vi "Calc Measruement Details.vi"(11 "Measurement properties":T1={"Measurement ID"=enum."1 signal, 1 ADC, 1 PJVS", "Description"="3 phase, 3 ADC, 1 PJVS", "Switching matrix M"=[], "Signal frequency  (Hz)"=50.0, "Maximal signal amplitude (V)"=0.0, "PRs (s)"=1.0, "PRe (s)"=50.0, "MRs (s)"=0.0, "MRe (s)"=0.0, "Set PJVS frequency (Hz)"=50.0, "PJVS reference voltages (1 period, V)"=[], "Requiested PJVS steps"=10, "Sampling f (Hz)"=0.0, "Trigger mode"=enum."Trigger every MX switch", "Timing matrix (periods)"=[], "Record length (multiples of M)"=1, "Calculated"={"Triggers to next path (line of sequence)"=[], "Record samples"=0, "Sample indexes of switches"=[], "PRs (samples)"=0, "PRe (samples)"=0, "MRs (samples)"=0, "MRe (samples)"=0, "Trigger frequency  (Hz)"=50.0, "Measurement druation (s)"=0.0, "Samples per step"=0.0, "QPMX Sequence"=[]}, "No of digitizers"=0, "No of transducers"=0, "Transducer corrections"=[]} {"Calculated"."Trigger frequency  (Hz)" format="%#_6p"; "Record length (multiples of M)" min=1 step=1; "PJVS reference voltages (1 period, V)" format="%.9g"; "MRe (s)" format="%#_4p"; "MRs (s)" format="%#_4p"; "PRe (s)" format="%#.4p"; "PRs (s)" format="%#_4p"}) -> (3 "Measurement properties out":T1={"Measurement ID"=enum."1 signal, 1 ADC, 1 PJVS", "Description"="3 phase, 3 ADC, 1 PJVS", "Switching matrix M"=[], "Signal frequency  (Hz)"=50.0, "Maximal signal amplitude (V)"=0.0, "PRs (s)"=1.0, "PRe (s)"=50.0, "MRs (s)"=0.0, "MRe (s)"=0.0, "Set PJVS frequency (Hz)"=50.0, "PJVS reference voltages (1 period, V)"=[], "Requiested PJVS steps"=10, "Sampling f (Hz)"=0.0, "Trigger mode"=enum."Trigger every MX switch", "Timing matrix (periods)"=[], "Record length (multiples of M)"=1, "Calculated"={"Triggers to next path (line of sequence)"=[], "Record samples"=0, "Sample indexes of switches"=[], "PRs (samples)"=0, "PRe (samples)"=0, "MRs (samples)"=0, "MRe (samples)"=0, "Trigger frequency  (Hz)"=50.0, "Measurement druation (s)"=0.0, "Samples per step"=0.0, "QPMX Sequence"=[]}, "No of digitizers"=0, "No of transducers"=0, "Transducer corrections"=[]} {"Calculated"."Trigger frequency  (Hz)" format="%#_6p"; "Record length (multiples of M)" min=1 step=1; "PJVS reference voltages (1 period, V)" format="%.9g"; "MRe (s)" format="%#_4p"; "MRs (s)" format="%#_4p"; "PRe (s)" format="%#.4p"; "PRs (s)" format="%#_4p"})   [LabVIEW 2020]
uses:
  Type definitions/Measuement properties.ctl
  Type definitions/Measurement ID.ctl
  Type definitions/Trigger mode.ctl
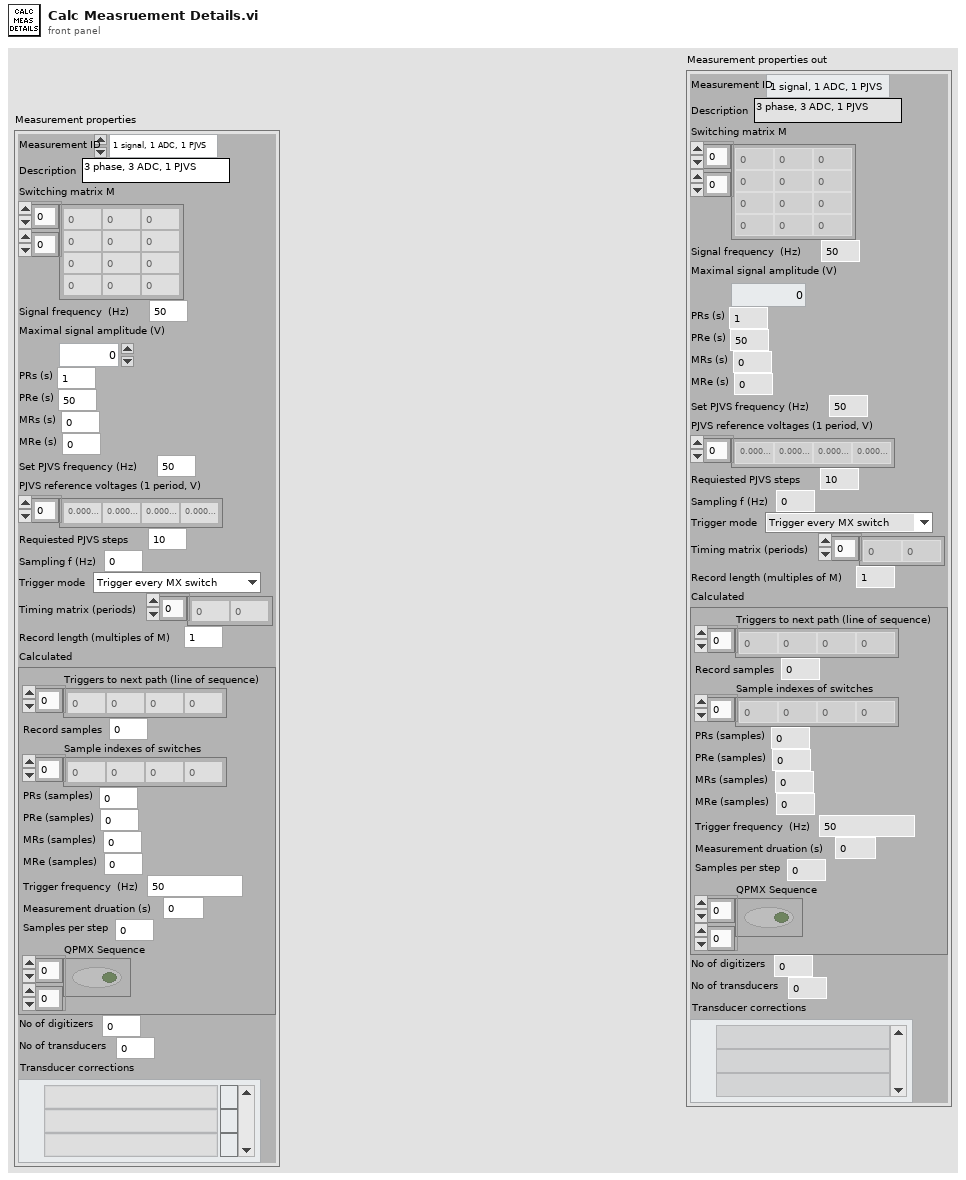
[diagram p1: front panel]
types:
  T1 = typedef "Measuement properties.ctl" = cluster{"Measurement ID":T2, "Description":string, "Switching matrix M":i32[][], "Signal frequency  (Hz)":dbl, "Maximal signal amplitude (V)":dbl, "PRs (s)":dbl, "PRe (s)":dbl, "MRs (s)":dbl, "MRe (s)":dbl, "Set PJVS frequency (Hz)":dbl, "PJVS reference voltages (1 period, V)":dbl[], "Requiested PJVS steps":u32, "Sampling f (Hz)":dbl, "Trigger mode":T3, "Timing matrix (periods)":i32[], "Record length (multiples of M)":u32, "Calculated":cluster{"Triggers to next path (line of sequence)":u32[], "Record samples":u32, "Sample indexes of switches":u32[], "PRs (samples)":i32, "PRe (samples)":i32, "MRs (samples)":i32, "MRe (samples)":i32, "Trigger frequency  (Hz)":dbl, "Measurement druation (s)":dbl, "Samples per step":dbl, "QPMX Sequence":bool[][]}, "No of digitizers":u32, "No of transducers":u32, "Transducer corrections":path[]}
  T2 = typedef "Measurement ID.ctl" = enum16{"Manual setup", "1 signal, 1 ADC, 1 PJVS", "1 phase (U, I), 1 ADC, 1 PJVS", "1 phase (U, I), 2 ADC, 1 PJVS", "1 phase (U, I), 3 ADC, 1 PJVS", "3 phases (U1..3, I1..3), 3 ADC, 1 PJVS"}
  T3 = typedef "Trigger mode.ctl" = enum16{"Trigger every MX switch", "Trigger every sample"}
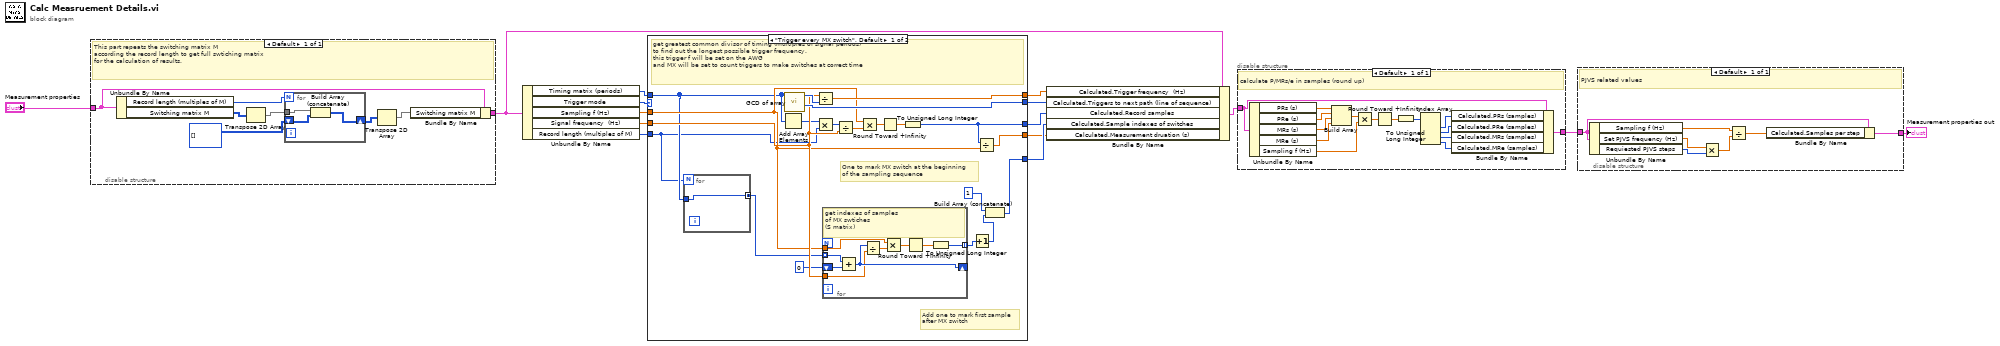
[diagram p0: block diagram]
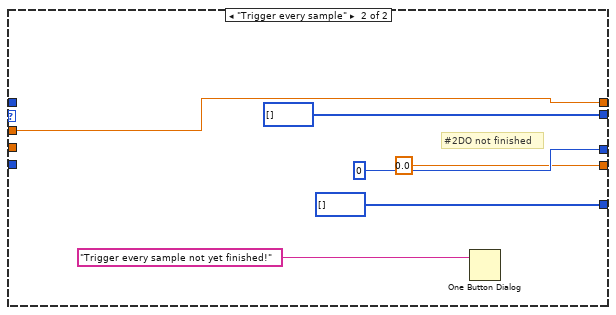
[diagram p2: hidden frame]
diagram:
  n1 = disable-structure shown="Default" {
    disable-tunnel: "Measurement properties" -> [w22]
    disable-tunnel: [w21] -> w1
    frame Enabled {
      # "This part repeats the switching matrix M\naccording the record length to get full swtiching matrix\nfor the calculation of results."
      n2 = Unbundle By Name(w22) -> ("Record length (multiples of M)"=w23:u32, "Switching matrix M"=w19:i32[][])
      n3 = Transpose 2D Array(2D array=w19) -> (transposed array=w18:i32[][])
      n4 = for {
        N: w23 -> [_]
        tunnel: w18 -> [w26]
        shift-right: [w24] -> w17
        shift-left: i32[][] [] ("Switching matrix M") -> [w25]
        n5 = Build Array (concatenate)(w26, w25) -> (w24:i32[][])
      }
      n6 = Transpose 2D Array(2D array=w17) -> (transposed array=w16:i32[][])
      n7 = Bundle By Name(cluster=w22, "Switching matrix M"=w16) -> (w21:T1)
    }
  }
  n8 = Unbundle By Name(w1) -> ("Timing matrix (periods)"=w7:i32[], "Trigger mode"=w15:T3, "Sampling f (Hz)"=w13:dbl, "Signal frequency  (Hz)"=w12:dbl, "Record length (multiples of M)"=w6:u32)
  n9 = case shown="\"Trigger every MX switch\", Default" w15 {
    tunnel: [w46 w62] -> w14
    tunnel: w13 -> [w36 w62]
    tunnel: w12 -> [w40 _]
    tunnel: w7 -> [w29 _]
    tunnel: [w44 u32[] [] ("Divisors")] -> w11
    tunnel: [w37 u32 0] -> w10
    tunnel: [w33 u32[] []] -> w9
    tunnel: w6 -> [w28 _]
    tunnel: [w35 0.0] -> w5
    frame "Trigger every MX switch", Default {
      # "Add one to mark first sample\nafter MX switch"
      # "One to mark MX switch at the beginning\nof the sampling sequence"
      # "get greatest common divisor of timing (multiples of signal periods)\nto find out the longest possible trigger frequency. \nthis trigger f will be set on the AWG\nand MX will be set to count triggers to make switches at correct time"
      n10 = for {
        N: w28 -> [_]
        tunnel: w29 -> [w47]
        tunnel: [w47] -> w27 mode=concatenating
      }
      n11 = Add Array Elements(numeric array=w29) -> (sum=w39:i32)
      n12 = call "GCD of array.vi"("Array"=w29) -> ("Divisors"=w44:u32[], "GCD"=w45:u32)  [unwired: 9 in]
      n13 = Divide(x=w40, y=w45) -> (x/y=w46:dbl)
      n14 = Multiply(x=w39, y=w28) -> (x*y=w38:u32)
      n15 = for {
        tunnel: w27 -> [w56] mode=indexing
        shift-right: [w51] -> _
        shift-left: u32 0 ("y") -> [w55]
        tunnel: w40 -> [w50]
        tunnel: [w49] -> w32 mode=indexing
        tunnel: w36 -> [w48]
        # "get indexes of samples\nof MX swtiches\n(S matrix)"
        n16 = Add(x=w56, y=w55) -> (x+y=w51:u32)
        n17 = Divide(x=w51, y=w50) -> (x/y=w52:dbl)
        n18 = Multiply(x=w48, y=w52) -> (x*y=w53:dbl)
        n19 = Round Toward +Infinity(x=w53) -> (ceil(x): smallest int >= x=w54:dbl)
        n20 = To Unsigned Long Integer(number=w54) -> (unsigned 32bit integer=w49:u32)
      }
      n21 = Divide(x=w38, y=w40) -> (x/y=w43:dbl)
      n22 = Multiply(x=w36, y=w43) -> (x*y=w42:dbl)
      n23 = Round Toward +Infinity(x=w42) -> (ceil(x): smallest int >= x=w41:dbl)
      n24 = To Unsigned Long Integer(number=w41) -> (unsigned 32bit integer=w37:u32)
      n25 = Increment(x=w32) -> (x+1=w31:u32[])
      n26 = Divide(x=w37, y=w36) -> (x/y=w35:dbl)
      n27 = Build Array (concatenate)(u32 1 ("y"), w31) -> (w33:u32[])
    }
    frame "Trigger every sample" {
      # "#2DO not finished"
      n28 = One Button Dialog(message="Trigger every sample not yet finished!") -> ()  [unwired: 1 in, 1 out]
    }
  }
  n29 = Bundle By Name(cluster=w1, "Calculated.Trigger frequency  (Hz)"=w14, "Calculated.Triggers to next path (line of sequence)"=w11, "Calculated.Record samples"=w10, "Calculated.Sample indexes of switches"=w9, "Calculated.Measurement druation (s)"=w5) -> (w8:T1)
  n30 = disable-structure shown="Default" {
    disable-tunnel: w8 -> [w63]
    disable-tunnel: [w64] -> w4
    frame Enabled {
      # "calculate P/MRs/e in samples (round up)"
      n31 = Unbundle By Name(w63) -> ("PRs (s)"=w77:dbl, "PRe (s)"=w76:dbl, "MRs (s)"=w75:dbl, "MRe (s)"=w74:dbl, "Sampling f (Hz)"=w73:dbl)
      n32 = Build Array(w77, w76, w75, w74) -> (w72:dbl[])
      n33 = Multiply(x=w72, y=w73) -> (x*y=w71:dbl[])
      n34 = Round Toward +Infinity(x=w71) -> (ceil(x): smallest int >= x=w70:dbl[])
      n35 = To Unsigned Long Integer(number=w70) -> (unsigned 32bit integer=w69:u32[])
      n36 = Index Array(array=w69) -> (element #1=w68:u32, element #2=w67:u32, element #3=w66:u32, element #4=w65:u32)  [unwired: 4 in]
      n37 = Bundle By Name(cluster=w63, "Calculated.PRs (samples)"=w68, "Calculated.PRe (samples)"=w67, "Calculated.MRs (samples)"=w66, "Calculated.MRe (samples)"=w65) -> (w64:T1)
    }
  }
  n38 = disable-structure shown="Default" {
    disable-tunnel: w4 -> [w79]
    disable-tunnel: [w80] -> w3
    frame Enabled {
      # "PJVS related values"
      n39 = Unbundle By Name(w79) -> ("Sampling f (Hz)"=w81:dbl, "Set PJVS frequency (Hz)"=w84:dbl, "Requiested PJVS steps"=w83:u32)
      n40 = Multiply(x=w84, y=w83) -> (x*y=w82:dbl)
      n41 = Divide(x=w81, y=w82) -> (x/y=w78:dbl)
      n42 = Bundle By Name(cluster=w79, "Calculated.Samples per step"=w78) -> (w80:T1)
    }
  }
  "Measurement properties out" <- w3
